vi "test-cubic-spline-05.vi"() -> ()   [LabVIEW 2019]
uses:
  <vilib>/Rock Robotics/WPI/ThirdParty/JAS_Junk/TrajLib/POSEwCURVATURE.ctl
  <vilib>/Rock Robotics/WPI/ThirdParty/JAS_Junk/TrajLib/POSE2D.ctl
  <vilib>/Rock Robotics/WPI/ThirdParty/JAS_Junk/TrajLib/TRANSLATION2D.ctl
  <vilib>/Rock Robotics/WPI/ThirdParty/JAS_Junk/TrajLib/ROTATION2D.ctl
  <vilib>/Rock Robotics/WPI/ThirdParty/JAS_Junk/TrajLib/Rotation_CreateAngle.vi
  <vilib>/Rock Robotics/WPI/ThirdParty/JAS_Junk/TrajLib/Util_CalcDist.vi
  <vilib>/Rock Robotics/WPI/ThirdParty/JAS_Junk/TrajLib/Trajectory_Library.lvlib
panel:
  out "All Interior \nwayPoints\nFound (True)":bool
  out "end rot = 0":dbl
  out "end y = 0":dbl
  out "end x = 0":dbl
  out "start rot = 0":dbl
  out "start y = 0":dbl
  out "start x = 0":dbl
  out "max dtheta < 0.0872":dbl
  out "max dy < 0.00127":dbl
  out "max dx  < 0.127":dbl
  out "Overall Error":errorcluster
  out "Elements":i32
  out "Create Spline Error":errorcluster
  out "SplinePoses\nWCurve":T1[](array[typedef]) {"POSE"."ROTATION"."SIN" format="%13.4f"; "POSE"."ROTATION"."COS" format="%13.4f"; "POSE"."ROTATION"."VALUE" format="%13.4f"; "POSE"."TRANSLATION"."Y" format="%14.3f"; "POSE"."TRANSLATION"."X" format="%14.3f"}
  out "Elapsed Time":dbl
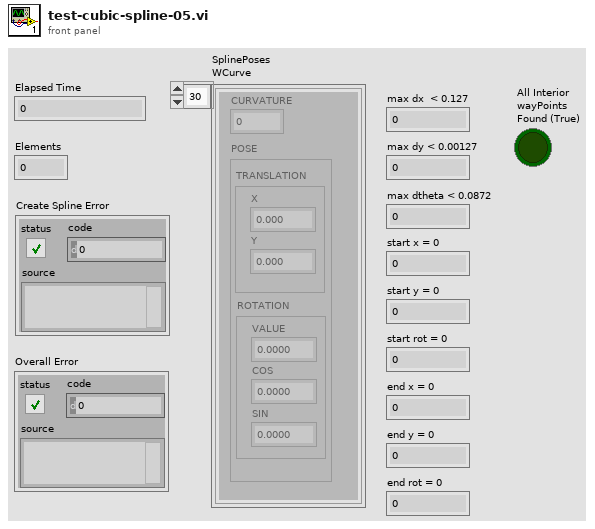
[diagram p1: front panel]
types:
  T1 = typedef "Trajectory_Library.lvlib/POSEwCURVATURE.ctl" = cluster{"CURVATURE":dbl, "POSE":T2}
  T2 = typedef "Trajectory_Library.lvlib/POSE2D.ctl" = cluster{"TRANSLATION":T3, "ROTATION":T4}
  T3 = typedef "Trajectory_Library.lvlib/TRANSLATION2D.ctl" = cluster{"X":dbl, "Y":dbl}
  T4 = typedef "Trajectory_Library.lvlib/ROTATION2D.ctl" = cluster{"VALUE":dbl, "COS":dbl, "SIN":dbl}
  T5 = typedef "Trajectory_Library.lvlib/SPLINE_CTRL_VECTOR.ctl" = cluster{"Xs":dbl[], "Ys":dbl[]}
  T6 = typedef "Trajectory_Library.lvlib/SPLINE.ctl" = cluster{"Degree":i32, "Coefficients":T7}
  T7 = typedef "NI_Matrix.lvlib/RealMatrix.ctl" = dbl[][]
  T8 = typedef "Trajectory_Library.lvlib/TWIST2D.ctl" = cluster{"dX":dbl, "dY":dbl, "dTHETA":dbl}
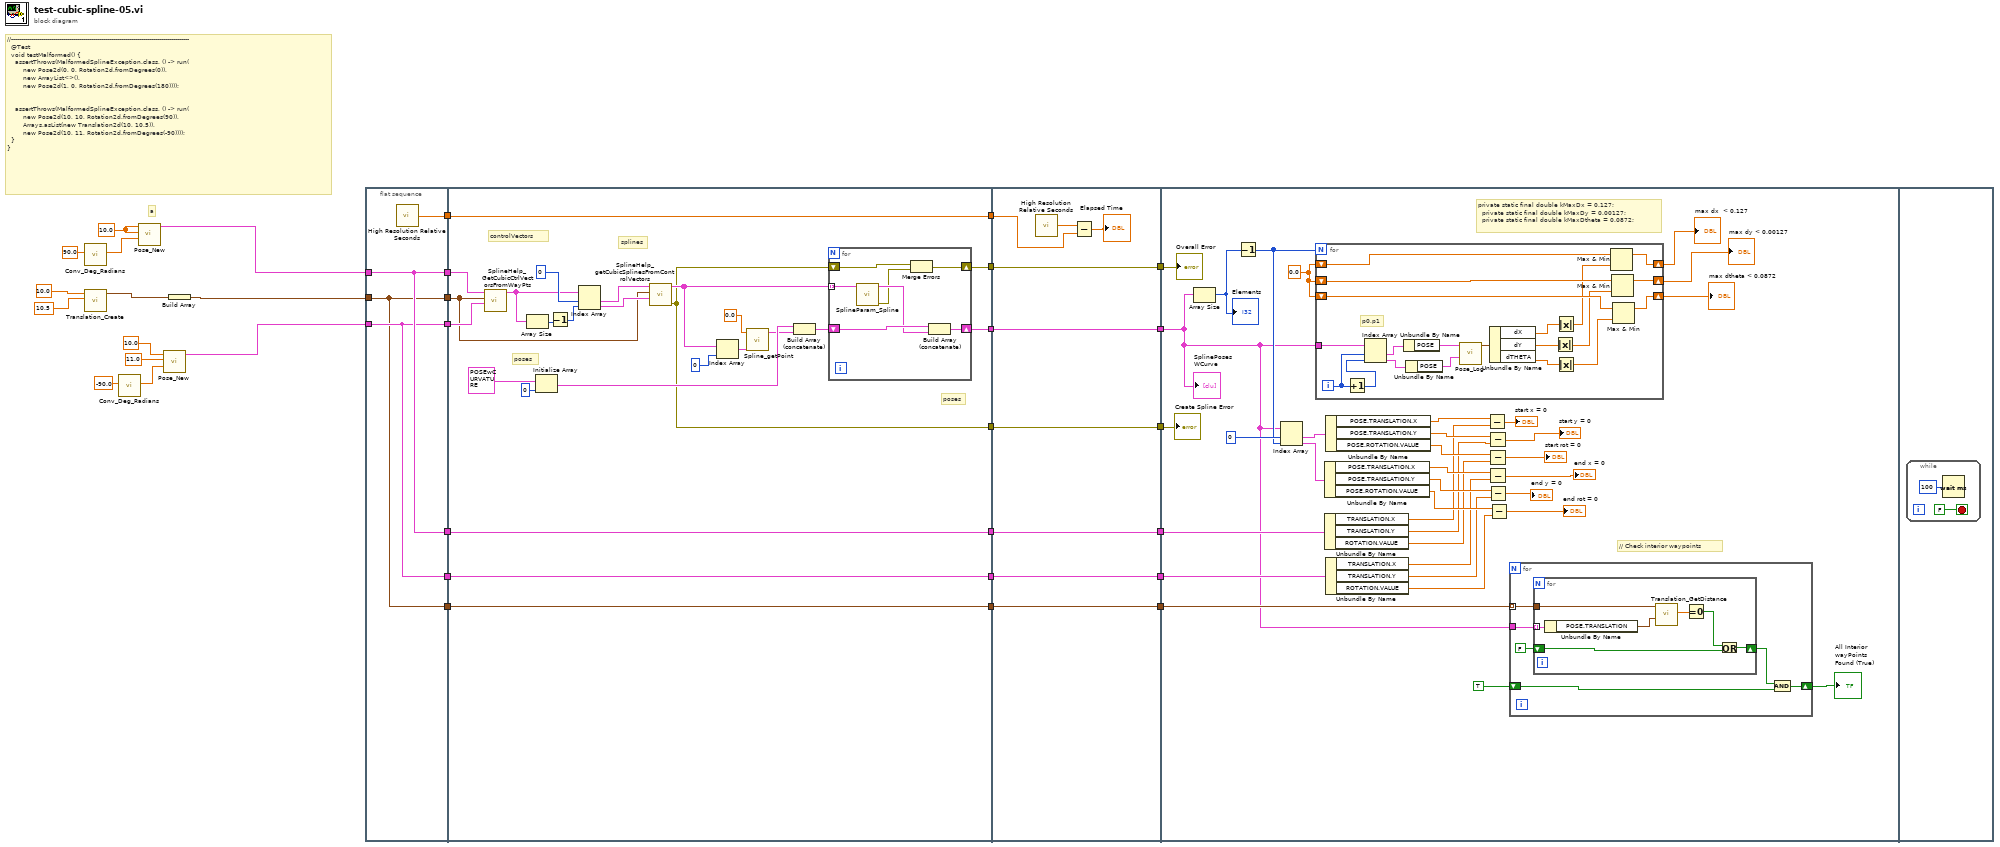
[diagram p0: block diagram]
diagram:
  w9 = 10.0 ("X")
  # "a"
  # "//-----------------------------------------------------------------------------------------\n  @Test\n  void testMalformed() {\n    assertThrows(MalformedSplineException.class, () -> run(\n        new Pose2d(0, 0, Rotation2d.fromDegrees(0)),\n        new ArrayList<>(), \n        new Pose2d(1, 0, Rotation2d.fromDegrees(180))));\n\n\n    assertThrows(MalformedSplineException.class, () -> run(\n        new Pose2d(10, 10, Rotation2d.fromDegrees(90)),\n        Arrays.asList(new Translation2d(10, 10.5)),\n        new Pose2d(10, 11, Rotation2d.fromDegrees(-90))));\n  }\n}"
  n1 = call <vilib>:"Conv_Deg_Radians.vi"("Degress"=90.0) -> ("Radians"=w8:dbl)  [unwired: 10 in]
  n2 = call <vilib>:"Translation_Create.vi"("Y"=10.5, "X"=10.0) -> ("TRANSLATION"=w1:T3)  [unwired: 9 in]
  n3 = call <vilib>:"Conv_Deg_Radians.vi"("Degress"=-90.0) -> ("Radians"=w5:dbl)  [unwired: 10 in]
  n4 = call <vilib>:"Pose_New.vi"("Heading"=w8, "Y"=w9, "X"=w9) -> ("out POSe"=w31:T2)  [unwired: 8 in]
  n5 = call <vilib>:"Pose_New.vi"("Heading"=w5, "Y"=11.0, "X"=10.0) -> ("out POSe"=w28:T2)  [unwired: 8 in]
  n6 = Build Array(w1) -> (w2:T3[])
  n7 = flat-sequence {
    tunnel: w31 -> [w36]
    tunnel: [w36] -> w30
    tunnel: w2 -> [w34]
    tunnel: [w34] -> w29
    tunnel: w28 -> [w35]
    tunnel: [w35] -> w27
    tunnel: [w37] -> w26
    tunnel: [w36] -> w18
    tunnel: [w35] -> w15
    tunnel: [w34] -> w10
    tunnel: w30 -> [w62]
    tunnel: w29 -> [w54]
    tunnel: w27 -> [w61]
    tunnel: [w53] -> w25
    tunnel: w26 -> [w53]
    tunnel: [w43] -> w24
    tunnel: [w42] -> w22
    tunnel: [w41] -> w20
    tunnel: w18 -> [w40]
    tunnel: [w40] -> w17
    tunnel: w15 -> [w39]
    tunnel: [w39] -> w14
    tunnel: [w38] -> w11
    tunnel: w10 -> [w38]
    tunnel: w25 -> [w78]
    tunnel: w24 -> [w77]
    tunnel: [w77] -> w23
    tunnel: w22 -> [w76]
    tunnel: [w76] -> w21
    tunnel: w20 -> [w75]
    tunnel: [w75] -> w19
    tunnel: w17 -> [w72]
    tunnel: [w72] -> w16
    tunnel: w14 -> [w71]
    tunnel: [w71] -> w13
    tunnel: [w70] -> w12
    tunnel: w11 -> [w70]
    tunnel: w23 -> [w81]
    tunnel: w21 -> [w113]
    tunnel: w19 -> [w112]
    tunnel: w16 -> [w106]
    tunnel: w13 -> [w105]
    tunnel: w12 -> [w82]
    frame #0 {
      n8 = call <vilib>:"High Resolution Relative Seconds.vi"() -> ("relative seconds"=w37:dbl)
    }
    frame #1 {
      # "poses"
      # "poses"
      # "splines"
      # "controlVectors"
      n9 = call <vilib>:"SplineHelp_GetCubicCtrlVectorsFromWayPts.vi"("Enging POSE"=w61, "Interior WAYPOINTS"=w54, "Starting POSE"=w62) -> ("SplineControlVectors"=w58:T5[])  [unwired: 8 in]
      n10 = Array Size(array=w58) -> (size(s)=w59:i32)
      n11 = Initialize Array(T1 {"CURVATURE"=0.0, "POSE"={"TRANSLATION"={"X"=0.0, "Y"=0.0}, "ROTATION"={"VALUE"=0.0, "COS"=1.0, "SIN"=0.0}}} ("POSEwCURVATURE"), 0 ("dimension size")) -> (w47:T1[])
      n12 = Decrement(x=w59) -> (x-1=w57:i32)
      n13 = Index Array(array=w58, index #1=0 ("index"), index #2=w57) -> (element #1=w56:T5, element #2=w55:T5)
      n14 = call <vilib>:"SplineHelp_getCubicSplinesFromControlVectors.vi"("endCtrlVector"=w55, "InternalWaypoints"=w54, "startCtrlVector"=w56) -> ("error out"=w42:errorcluster, "splines"=w44:T6[])  [unwired: 3 in, 4 out]
      n15 = Index Array(array=w44, index=0) -> (element=w49:T6)
      n16 = call <vilib>:"Spline_getPoint.vi"("inputSPLINE"=w49, "Time"=0.0) -> ("POSEwCURVATURE"=w46:T1)  [unwired: 9 in]
      n17 = Build Array (concatenate)(w47, w46) -> (w45:T1[])
      n18 = for {
        shift-right: [w66] -> w43
        shift-left: w45 -> [w68]
        tunnel: w44 -> [w69] mode=indexing
        shift-right: [w64] -> w41
        shift-left: w42 -> [w65]
        n19 = call <vilib>:"SplineParam_Spline.vi"("inputSPLINE"=w69) -> ("error out"=w63:errorcluster, "outputPOSEwCURVATURE"=w67:T1[])  [unwired: 9 in]
        n20 = Merge Errors(w65, w63) -> (w64:errorcluster)
        n21 = Build Array (concatenate)(w68, w67) -> (w66:T1[])
      }
    }
    frame #2 {
      n22 = call <vilib>:"High Resolution Relative Seconds.vi"() -> ("relative seconds"=w73:dbl)
      n23 = Subtract(x=w73, y=w78) -> (x-y=→"Elapsed Time":dbl)
    }
    frame #3 {
      w110 = 0.0
      # "// Check interior waypoints"
      # "private static final double kMaxDx = 0.127;\n  private static final double kMaxDy = 0.00127;\n  private static final double kMaxDtheta = 0.0872;"
      n24 = Array Size(array=w81) -> (size(s)=w111:i32)
      "Elements" <- w111
      n25 = Decrement(x=w111) -> (x-1=w103:i32)
      n26 = Index Array(array=w81, index #1=0 ("index"), index #2=w103) -> (element #1=w102:T1, element #2=w101:T1)
      n27 = for {
        N: w103 -> [_]
        tunnel: w81 -> [w144]
        shift-right: [w135] -> w109
        shift-left: w110 -> [w132]
        shift-right: [w133] -> w107
        shift-left: w110 -> [w130]
        shift-right: [w134] -> w108
        shift-left: w110 -> [w131]
        i -> [w146]
        # "p0,p1"
        n28 = Increment(x=w146) -> (x+1=w145:i32)
        n29 = Index Array(array=w144, index #1=w146, index #2=w145) -> (element #1=w143:T1, element #2=w142:T1)
        n30 = Unbundle By Name(w143) -> ("POSE"=w141:T2)
        n31 = Unbundle By Name(w142) -> ("POSE"=w140:T2)
        n32 = call <vilib>:"Pose_Log.vi"("end POSE"=w140, "in POSE"=w141) -> ("out TWIST"=w139:T8)  [unwired: 9 in]
        n33 = Unbundle By Name(w139) -> ("dX"=w136:dbl, "dY"=w137:dbl, "dTHETA"=w138:dbl)
        n34 = Absolute Value(x=w137) -> (abs(x)=w128:dbl)
        n35 = Absolute Value(x=w136) -> (abs(x)=w129:dbl)
        n36 = Absolute Value(x=w138) -> (abs(x)=w127:dbl)
        n37 = Max & Min(x=w132, y=w129) -> (max(x,y)=w135:dbl)  [unwired: 1 out]
        n38 = Max & Min(x=w131, y=w128) -> (max(x,y)=w134:dbl)  [unwired: 1 out]
        n39 = Max & Min(x=w130, y=w127) -> (max(x,y)=w133:dbl)  [unwired: 1 out]
      }
      "max dx  < 0.127" <- w109
      "max dy < 0.00127" <- w108
      "max dtheta < 0.0872" <- w107
      n40 = Unbundle By Name(w101) -> ("POSE.TRANSLATION.X"=w97:dbl, "POSE.TRANSLATION.Y"=w96:dbl, "POSE.ROTATION.VALUE"=w95:dbl)
      n41 = Unbundle By Name(w106) -> ("TRANSLATION.X"=w94:dbl, "TRANSLATION.Y"=w93:dbl, "ROTATION.VALUE"=w92:dbl)
      n42 = Unbundle By Name(w102) -> ("POSE.TRANSLATION.X"=w100:dbl, "POSE.TRANSLATION.Y"=w99:dbl, "POSE.ROTATION.VALUE"=w98:dbl)
      n43 = Unbundle By Name(w105) -> ("TRANSLATION.X"=w91:dbl, "TRANSLATION.Y"=w90:dbl, "ROTATION.VALUE"=w89:dbl)
      n44 = Subtract(x=w100, y=w94) -> (x-y=→"start x = 0":dbl)
      n45 = Subtract(x=w99, y=w93) -> (x-y=→"start y = 0":dbl)
      n46 = Subtract(x=w98, y=w92) -> (x-y=→"start rot = 0":dbl)
      n47 = Subtract(x=w97, y=w91) -> (x-y=→"end x = 0":dbl)
      n48 = Subtract(x=w96, y=w90) -> (x-y=→"end y = 0":dbl)
      n49 = Subtract(x=w95, y=w89) -> (x-y=→"end rot = 0":dbl)
      n50 = for {
        tunnel: w82 -> [w114] mode=indexing
        tunnel: w81 -> [w119]
        shift-right: [w118] -> w79
        shift-left: TRUE -> [w117]
        n51 = for {
          tunnel: w119 -> [w123] mode=indexing
          shift-right: [w126] -> w115
          shift-left: FALSE -> [w125]
          tunnel: w114 -> [w124]
          n52 = Unbundle By Name(w123) -> ("POSE.TRANSLATION"=w122:T3)
          n53 = call <vilib>:"Translation_GetDistance.vi"("other Translation"=w122, "In Translation"=w124) -> ("Distance"=w121:dbl)  [unwired: 9 in]
          n54 = Equal To 0?(x=w121) -> (x = 0?=w120:bool)
          n55 = Or(x=w120, y=w125) -> (x .or. y?=w126:bool)
        }
        n56 = And(x=w115, y=w117) -> (x .and. y?=w118:bool)
      }
      "All Interior \nwayPoints\nFound (True)" <- w79
      "SplinePoses\nWCurve" <- w81
      "Create Spline Error" <- w113
      "Overall Error" <- w112
    }
    frame #4 {
      n57 = while {
        stop <- FALSE stop-if-true
        n58 = Wait (ms)(milliseconds to wait=u32 100) -> ()  [unwired: 1 out]
      }
    }
  }
